vi "Init Module Init Queue.vi"(11 "Strings[]":string[](array[string])) -> (3 "Queue out":refnum<queue>)   [LabVIEW 2020]
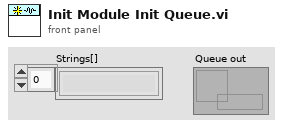
[diagram p1: front panel]
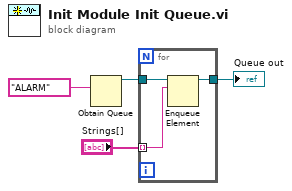
[diagram p0: block diagram]
diagram:
  n1 = Obtain Queue(element data type="ALARM" ("Combo Box")) -> (queue out=w3:refnum<queue>)  [unwired: 4 in, 2 out]
  n2 = for {
    tunnel: "Strings[]" -> [w7] mode=indexing
    tunnel: w3 -> [w6]
    tunnel: [w5] -> w4
    n3 = Enqueue Element(queue=w6, element=w7) -> (queue out=w5:refnum<queue>)  [unwired: 2 in, 2 out]
  }
  "Queue out" <- w4
